vi "Get Broadcast Event.vi"(8 "error in (no error)":errorcluster, 11 "Process in":refnum<class "Process.lvclass">) -> (0 "error out":errorcluster, 2 "Broadcast Event":refnum<user-event>[](array[refnum]), 3 "Process out":refnum<class "Process.lvclass">)   [LabVIEW 2020, in "Process.lvclass"]
doc: "Get the broadcast event used to send broadcasts to registered observers."
uses:
  Process.lvclass
  Protected/Broadcasting/Broadcast Message Cluster.ctl
  Process.lvclass/Process.ctl
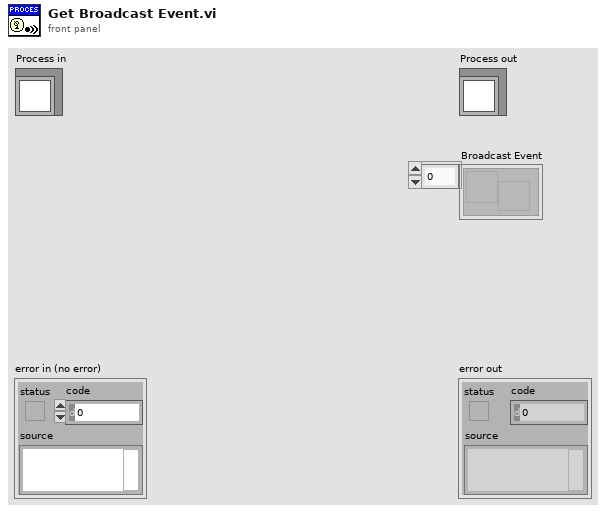
[diagram p1: front panel]
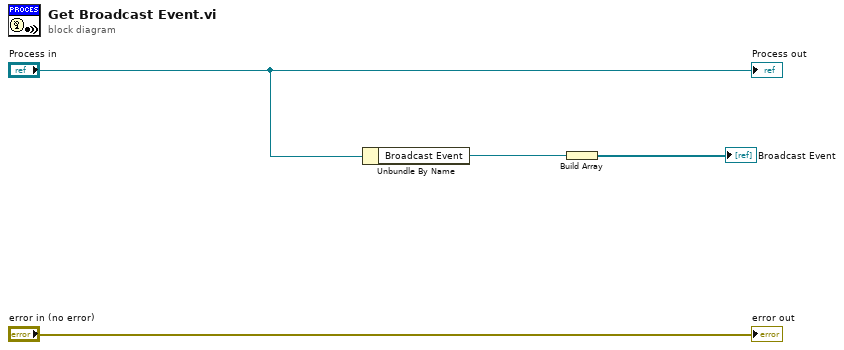
[diagram p0: block diagram]
diagram:
  n1 = Unbundle By Name("Process in") -> ("Broadcast Event"=w2:refnum<user-event>)
  n2 = Build Array(w2) -> (→"Broadcast Event":refnum<user-event>[])
  "error out" <- "error in (no error)"
  "Process out" <- "Process in"
